vi "Capture_Flow_Vis.vi"(3 "Mode":T5, 5 "Traverse line In":T2 {"Carrier_2 Q (l/min)" format="%#.2f"; "Row Duration (mins)" format="%#.1f"; "Row No" min=0; "Trace Gas Concentration (%)" min=0.0 format="%#_4f"; "Carrier_1 Q (l/min)" format="%#.2f"; "Tunnel Speed" format="%#.2f"; "Start X" format="%#.2f"; "Start Y" format="%#.2f"; "Start Z" format="%#.2f"; "End X" format="%#.2f"; "End Y" format="%#.2f"; "End Z" format="%#.2f"; "Averaging time (min)" min=0.0 format="%#.2f"}) -> (0 "Error Message":string, 1 "Status":T1, 2 "Traverse line Out":T2 {"Carrier_2 Q (l/min)" format="%#.2f"; "Row Duration (mins)" format="%#.1f"; "Row No" min=0; "Trace Gas Concentration (%)" min=0.0 format="%#_4f"; "Carrier_1 Q (l/min)" format="%#.2f"; "Tunnel Speed" format="%#.2f"; "Start X" format="%#.2f"; "Start Y" format="%#.2f"; "Start Z" format="%#.2f"; "End X" format="%#.2f"; "End Y" format="%#.2f"; "End Z" format="%#.2f"; "Averaging time (min)" min=0.0 format="%#.2f"})   [LabVIEW 2015]
uses:
  Gen Trav/Traverse_cluster.ctl
  Gen Trav/Spacing.ctl
  Controls/Multi_run_mode.ctl
  Controls/User_Specific_mode.ctl
  Gen Trav/Multi_Run_Status.ctl
  ADAM Client/Sub VIs/ADAM Controls/Update_scan_value.ctl
  Controls/Setup.ctl
  Controls/Save_Data.ctl
  Globals/Extra_Commands_Global.vi
  Globals/Meas_global.vi
panel:
  in  "Enable smoke time (Sec)":dbl=3.0
  # "X           Y            Z"
  # "Start"
  # "End"
  # "X           Y            Z"
  # "Start"
  # "End"
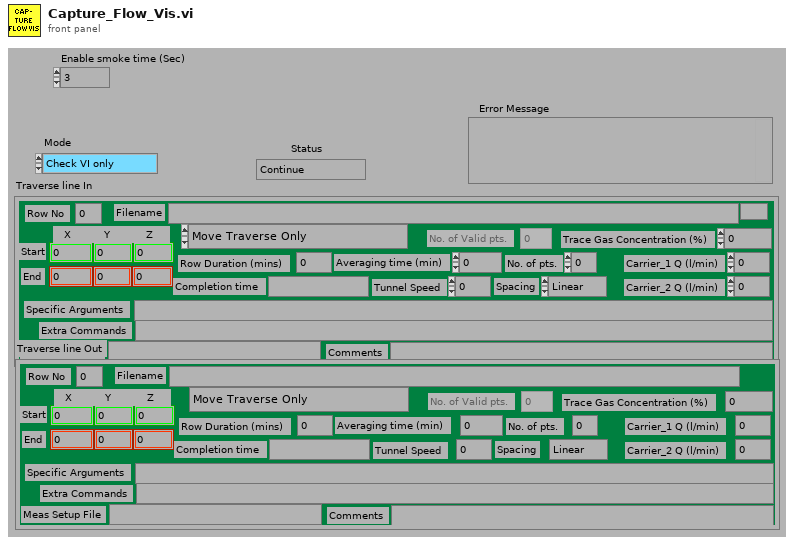
[diagram p1: front panel]
types:
  T1 = typedef "Multi_Run_Status.ctl" = enum16{"Continue", "Jump to Next Point", "Jump to Next Row", "Jump To Fall Back", "Terminate Run"}
  T2 = typedef "Traverse_cluster.ctl" = cluster{"Start X":sgl, "Start Y":sgl, "Start Z":sgl, "End X":sgl, "End Y":sgl, "End Z":sgl, "No. of pts.":i32, "Spacing":T3, "Filename":path, "Tunnel Speed":dbl, "Averaging time (min)":dbl, "Extra Commands":string, "Carrier_1 Q (l/min)":dbl, "Carrier_2 Q (l/min)":dbl, "Trace Gas Concentration (%)":dbl, "Specific Arguments":string, "Comments":string, "Row No":i32, "Row Type Selector":T4, "Completion time":string, "Row Duration (mins)":dbl, "No. of Valid pts.":i32, "Meas Setup File":string}
  T3 = typedef "Spacing.ctl" = enum16{"Linear", "Log", "Gauss", "Specified", "N/A"}
  T4 = typedef "Multi_run_mode.ctl" = enum16{"Move Traverse Only", "Set Tunnel Speed Only", "Set Source Only", "Set Measurement Conditions", "Single Measurement", "Vertical Profile", "Lateral Profile", "Longitudinal Profile", "Explore Volume", "Multi-Axis Profile", "Auto Calibrate", "Meas Fast FID Bkgnd", "Check Beam Power", "Scanning Valve Measurement", "Run VI Named:", "Set ADAM Ch", "Wait (minutes)", "Send Message", "Synchronize With:", "Fall Back to this Row", "Turn Off Row Repeating", "Blank Row", "Traverse 3D Volume"}
  T5 = typedef "User_Specific_mode.ctl" = enum16{"Check VI only", "Run VI"}
  T6 = typedef "Update_scan_value.ctl" = cluster{"Channel Name":string, "New Value":dbl}
  T7 = typedef "Save_Data.ctl" = enum16{"Save No Data", "Save Data"}
  T8 = typedef "Setup.ctl" = enum16{"Run Program", "Show Setup", "Save Current Setup", "Setup Front Panel"}
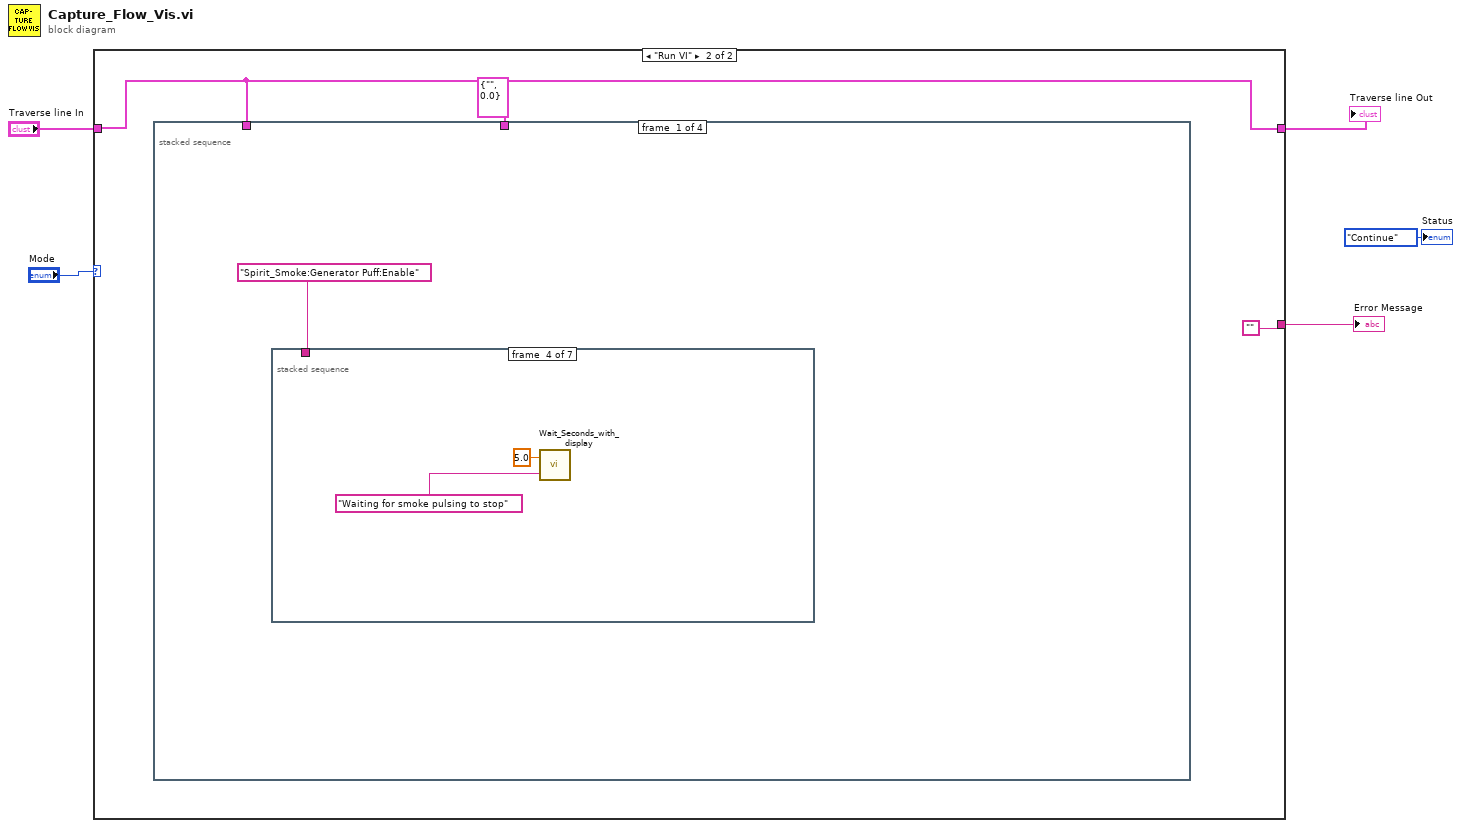
[diagram p0: block diagram]
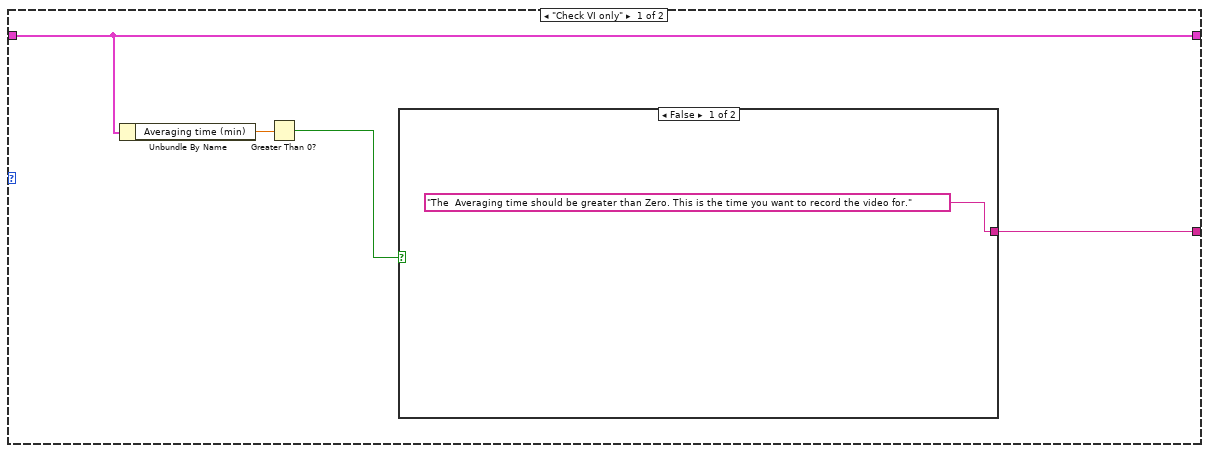
[diagram p2: hidden frame]
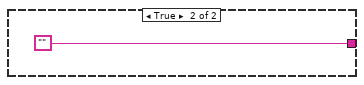
[diagram p3: hidden frame]
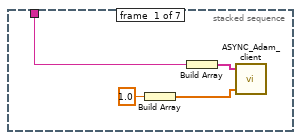
[diagram p4: hidden frame]
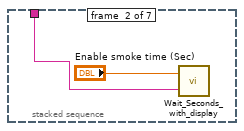
[diagram p5: hidden frame]
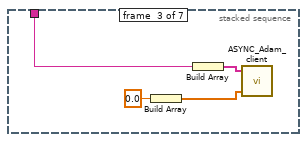
[diagram p6: hidden frame]
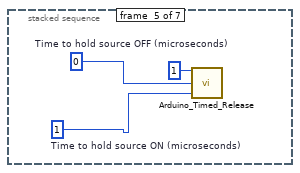
[diagram p7: hidden frame]
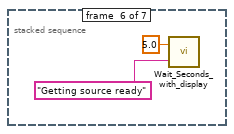
[diagram p8: hidden frame]
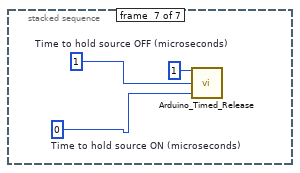
[diagram p9: hidden frame]
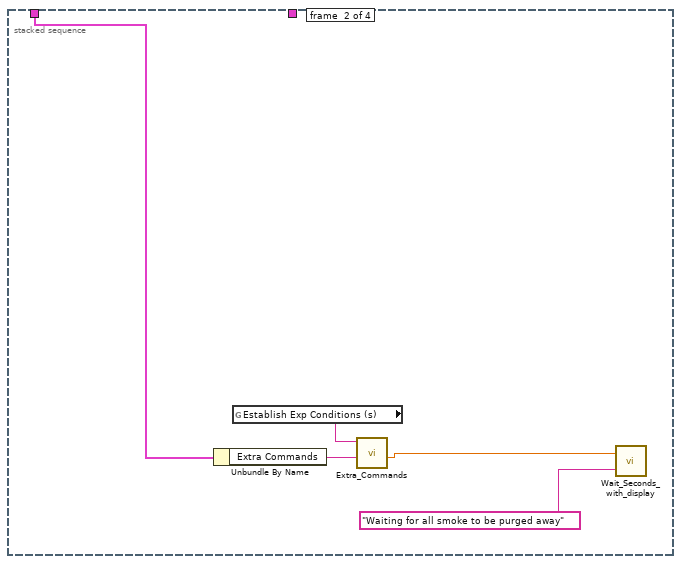
[diagram p10: hidden frame]
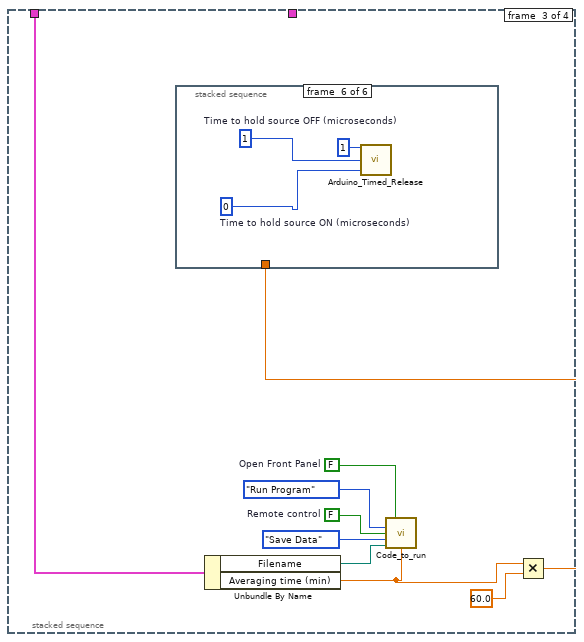
[diagram p11: hidden frame]
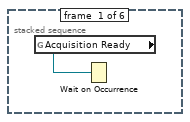
[diagram p12: hidden frame]
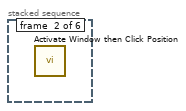
[diagram p13: hidden frame]
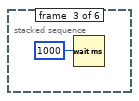
[diagram p14: hidden frame]
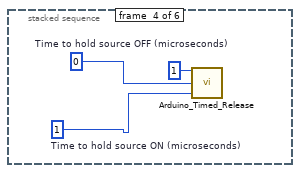
[diagram p15: hidden frame]
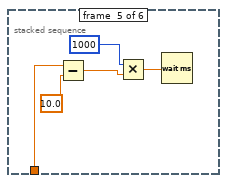
[diagram p16: hidden frame]
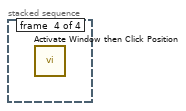
[diagram p17: hidden frame]
diagram:
  n1 = case shown="\"Run VI\"" "Mode" {
    tunnel: "Traverse line In" -> [w8 w12]
    tunnel: [w8 w12] -> w3
    tunnel: [w9 ""] -> w2
    frame "Check VI only" {
      n2 = Unbundle By Name(w8) -> ("Averaging time (min)"=w7:dbl)
      n3 = Greater Than 0?(x=w7) -> (x > 0?=w6:bool)
      n4 = case shown="False" w6 {
        tunnel: ["The  Averaging time should be greater than Zero. This is the time you want to record the video for." ""] -> w9
        frame False {
        }
        frame True {
        }
      }
    }
    frame "Run VI" {
      n5 = stacked-sequence {
        tunnel: T6 {"Channel Name"="", "New Value"=0.0} ("Update Scan Value Cluster") -> [_ _ _ _]
        tunnel: w12 -> [_ w37 w49 _]
        frame #0 {
          n6 = stacked-sequence {
            tunnel: "Spirit_Smoke:Generator Puff:Enable" -> [w16 w20 w22 _ _ _ _]
            frame #0 {
              n7 = Build Array(1.0 ("element")) -> (w18:dbl[])
              n8 = Build Array(w16) -> (w19:string[])
              n9 = call "ASYNC_Adam_client.vi"("Values"=w18, "Channel Names"=w19) -> ()  [unwired: 1 in, 2 out]
            }
            frame #1 {
              n10 = call "Wait_Seconds_with_display.vi"("Message"=w20, "Seconds to wait"="Enable smoke time (Sec)") -> ()  [unwired: 1 in, 1 out]
            }
            frame #2 {
              n11 = Build Array(0.0 ("element")) -> (w24:dbl[])
              n12 = Build Array(w22) -> (w23:string[])
              n13 = call "ASYNC_Adam_client.vi"("Values"=w24, "Channel Names"=w23) -> ()  [unwired: 1 in, 2 out]
            }
            frame #3 {
              n14 = call "Wait_Seconds_with_display.vi"("Message"="Waiting for smoke pulsing to stop", "Seconds to wait"=5.0) -> ()  [unwired: 2 out]
            }
            frame #4 {
              w28 = u32 0  # Time to hold source OFF (microseconds)
              w29 = u32 1  # Time to hold source ON (microseconds)
              n15 = call "Arduino_Timed_Release.vi"("Time to hold source ON (microseconds)"=w29, "Time to hold source OFF (microseconds)"=w28, "Number of cycles"=u16 1) -> ()  [unwired: 2 out]
            }
            frame #5 {
              n16 = call "Wait_Seconds_with_display.vi"("Message"="Getting source ready", "Seconds to wait"=5.0) -> ()  [unwired: 2 out]
            }
            frame #6 {
              w33 = u32 1  # Time to hold source OFF (microseconds)
              w34 = u32 0  # Time to hold source ON (microseconds)
              n17 = call "Arduino_Timed_Release.vi"("Time to hold source ON (microseconds)"=w34, "Time to hold source OFF (microseconds)"=w33, "Number of cycles"=u16 1) -> ()  [unwired: 2 out]
            }
          }
        }
        frame #1 {
          n18 = Unbundle By Name(w37) -> ("Extra Commands"=w39:string)
          n19 = global read "Extra_Commands_Global.vi" "Establish Exp Conditions (s)"() -> (w38:string)
          n20 = call "Extra_Commands.vi"("String to Search"=w39, "Command"=w38) -> ("Numeric Value"=w36:dbl)  [unwired: 1 in, 4 out]
          n21 = call "Wait_Seconds_with_display.vi"("Message"="Waiting for all smoke to be purged away", "Seconds to wait"=w36) -> ()  [unwired: 1 in, 1 out]
        }
        frame #2 {
          w46 = FALSE  # Open Front Panel
          w47 = FALSE  # Remote control
          n22 = Unbundle By Name(w49) -> ("Filename"=w48:path, "Averaging time (min)"=w43:dbl)
          n23 = call "Code_to_run.vi"("Open Front Panel"=w46, "setup"=Setup."Run Program", "Remote control"=w47, "File"=Save_Data."Save Data", "Results Filename"=w48, "Averaging time (min)"=w43) -> ()  [unwired: 5 in, 5 out]
          n24 = Multiply(x=w43, y=60.0) -> (x*y=w41:dbl)
          n25 = stacked-sequence {
            tunnel: w41 -> [_ _ _ _ w59 _]
            frame #0 {
              n26 = global read "Meas_global.vi" "Acquisition Ready"() -> (w50:refnum<k4>)
              n27 = Wait on Occurrence(2:w50) -> ()  [unwired: 2 in, 1 out]
            }
            frame #1 {
              n28 = call "Activate Window then Click Position.vi"() -> ()  [unwired: 12 in]
            }
            frame #2 {
              n29 = Wait (ms)(milliseconds to wait=u32 1000 ("millisecond timer value")) -> ()  [unwired: 1 out]
            }
            frame #3 {
              w52 = u32 0  # Time to hold source OFF (microseconds)
              w53 = u32 1  # Time to hold source ON (microseconds)
              n30 = call "Arduino_Timed_Release.vi"("Time to hold source ON (microseconds)"=w53, "Time to hold source OFF (microseconds)"=w52, "Number of cycles"=u16 1) -> ()  [unwired: 2 out]
            }
            frame #4 {
              n31 = Subtract(x=w59, y=10.0) -> (x-y=w57:dbl)
              n32 = Multiply(x=u32 1000 ("millisecond timer value"), y=w57) -> (x*y=w55:dbl)
              n33 = Wait (ms)(milliseconds to wait=w55) -> ()  [unwired: 1 out]
            }
            frame #5 {
              w60 = u32 1  # Time to hold source OFF (microseconds)
              w61 = u32 0  # Time to hold source ON (microseconds)
              n34 = call "Arduino_Timed_Release.vi"("Time to hold source ON (microseconds)"=w61, "Time to hold source OFF (microseconds)"=w60, "Number of cycles"=u16 1) -> ()  [unwired: 2 out]
            }
          }
        }
        frame #3 {
          n35 = call "Activate Window then Click Position.vi"() -> ()  [unwired: 12 in]
        }
      }
    }
  }
  "Traverse line Out" <- w3
  "Error Message" <- w2
  "Status" <- Multi_Run_Status."Continue" ("Status")
